vi "PLC ModbusTest.vi"() -> ()   [LabVIEW 2019]
uses:
  <vilib>/Plasmionique/MB Master/MB_Master_TCP/MB_Master_TCP.lvclass
  <vilib>/NI/Modbus Library/API/Wrapper/API Main.lvlib
  <vilib>/NI/Modbus Library/API/Master/Modbus Master.lvclass
  <vilib>/NI/Modbus Library/API/Wrapper/Create TCP Master.vi
panel:
  out "register values 3":u16[](array[numeric])
  out "remote port 2":u16
  out "remote address 2":string
  out "listener ID out":refnum<k5>
  out "remote port":u16
  out "remote address":string
  out "Words":i16[](array[numeric])
  out "Information out":T1 {"Unit identifier" max=247; "exceptionCode" max=247}
  out "error out 5":errorcluster
  out "register values 2":u16[](array[numeric])
  out "register values":u16[](array[numeric])
  out "error out 4":errorcluster
  out "Registers":u16[](array[numeric])
  out "concatenated string":string
  in  "Input ASCII":string="A"
  out "hex integer string":string
  in  "string":string="WR ZF0.H 41\r"
  out "value":i32
  out "ASCII Output":string
  out "error out 2":errorcluster
  out "data out 4":string
  out "data out 3":string
  in  "timeout ms (60000) 2":i32=6000
  out "data out":string
  in  "String":string="RDS DM0 4\r"
  out "error out":errorcluster
  in  "timeout ms (60000)":i32=6000
  # "Input ASCII"
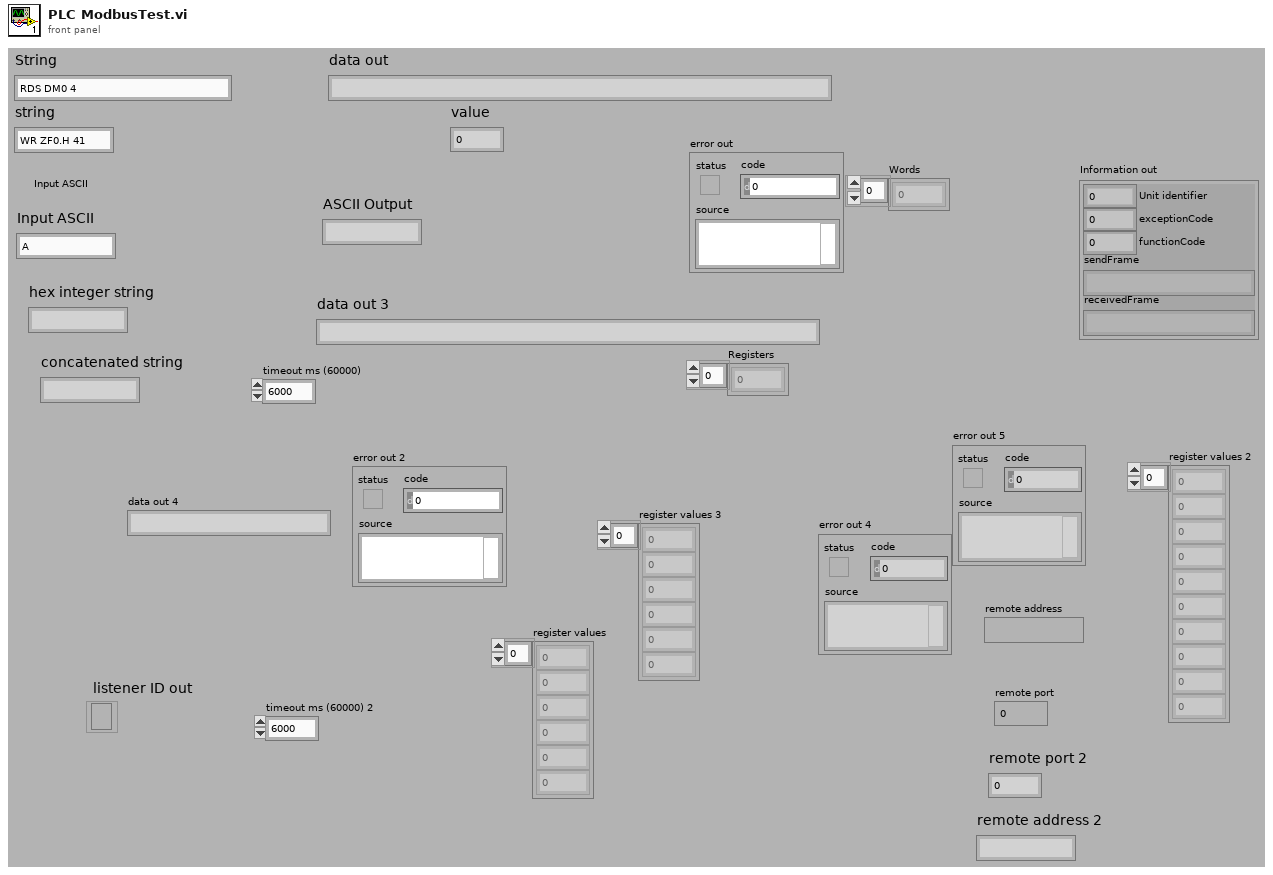
[diagram p1: front panel]
types:
  T1 = cluster{"Unit identifier":u8, "exceptionCode":u8, "functionCode":u8, "sendFrame":string, "receivedFrame":string}
  T2 = cluster{"server address":string, "remote port (502)":u16}
  T3 = enum16{"Standard", "Buffered", "CRLF", "Immediate"}
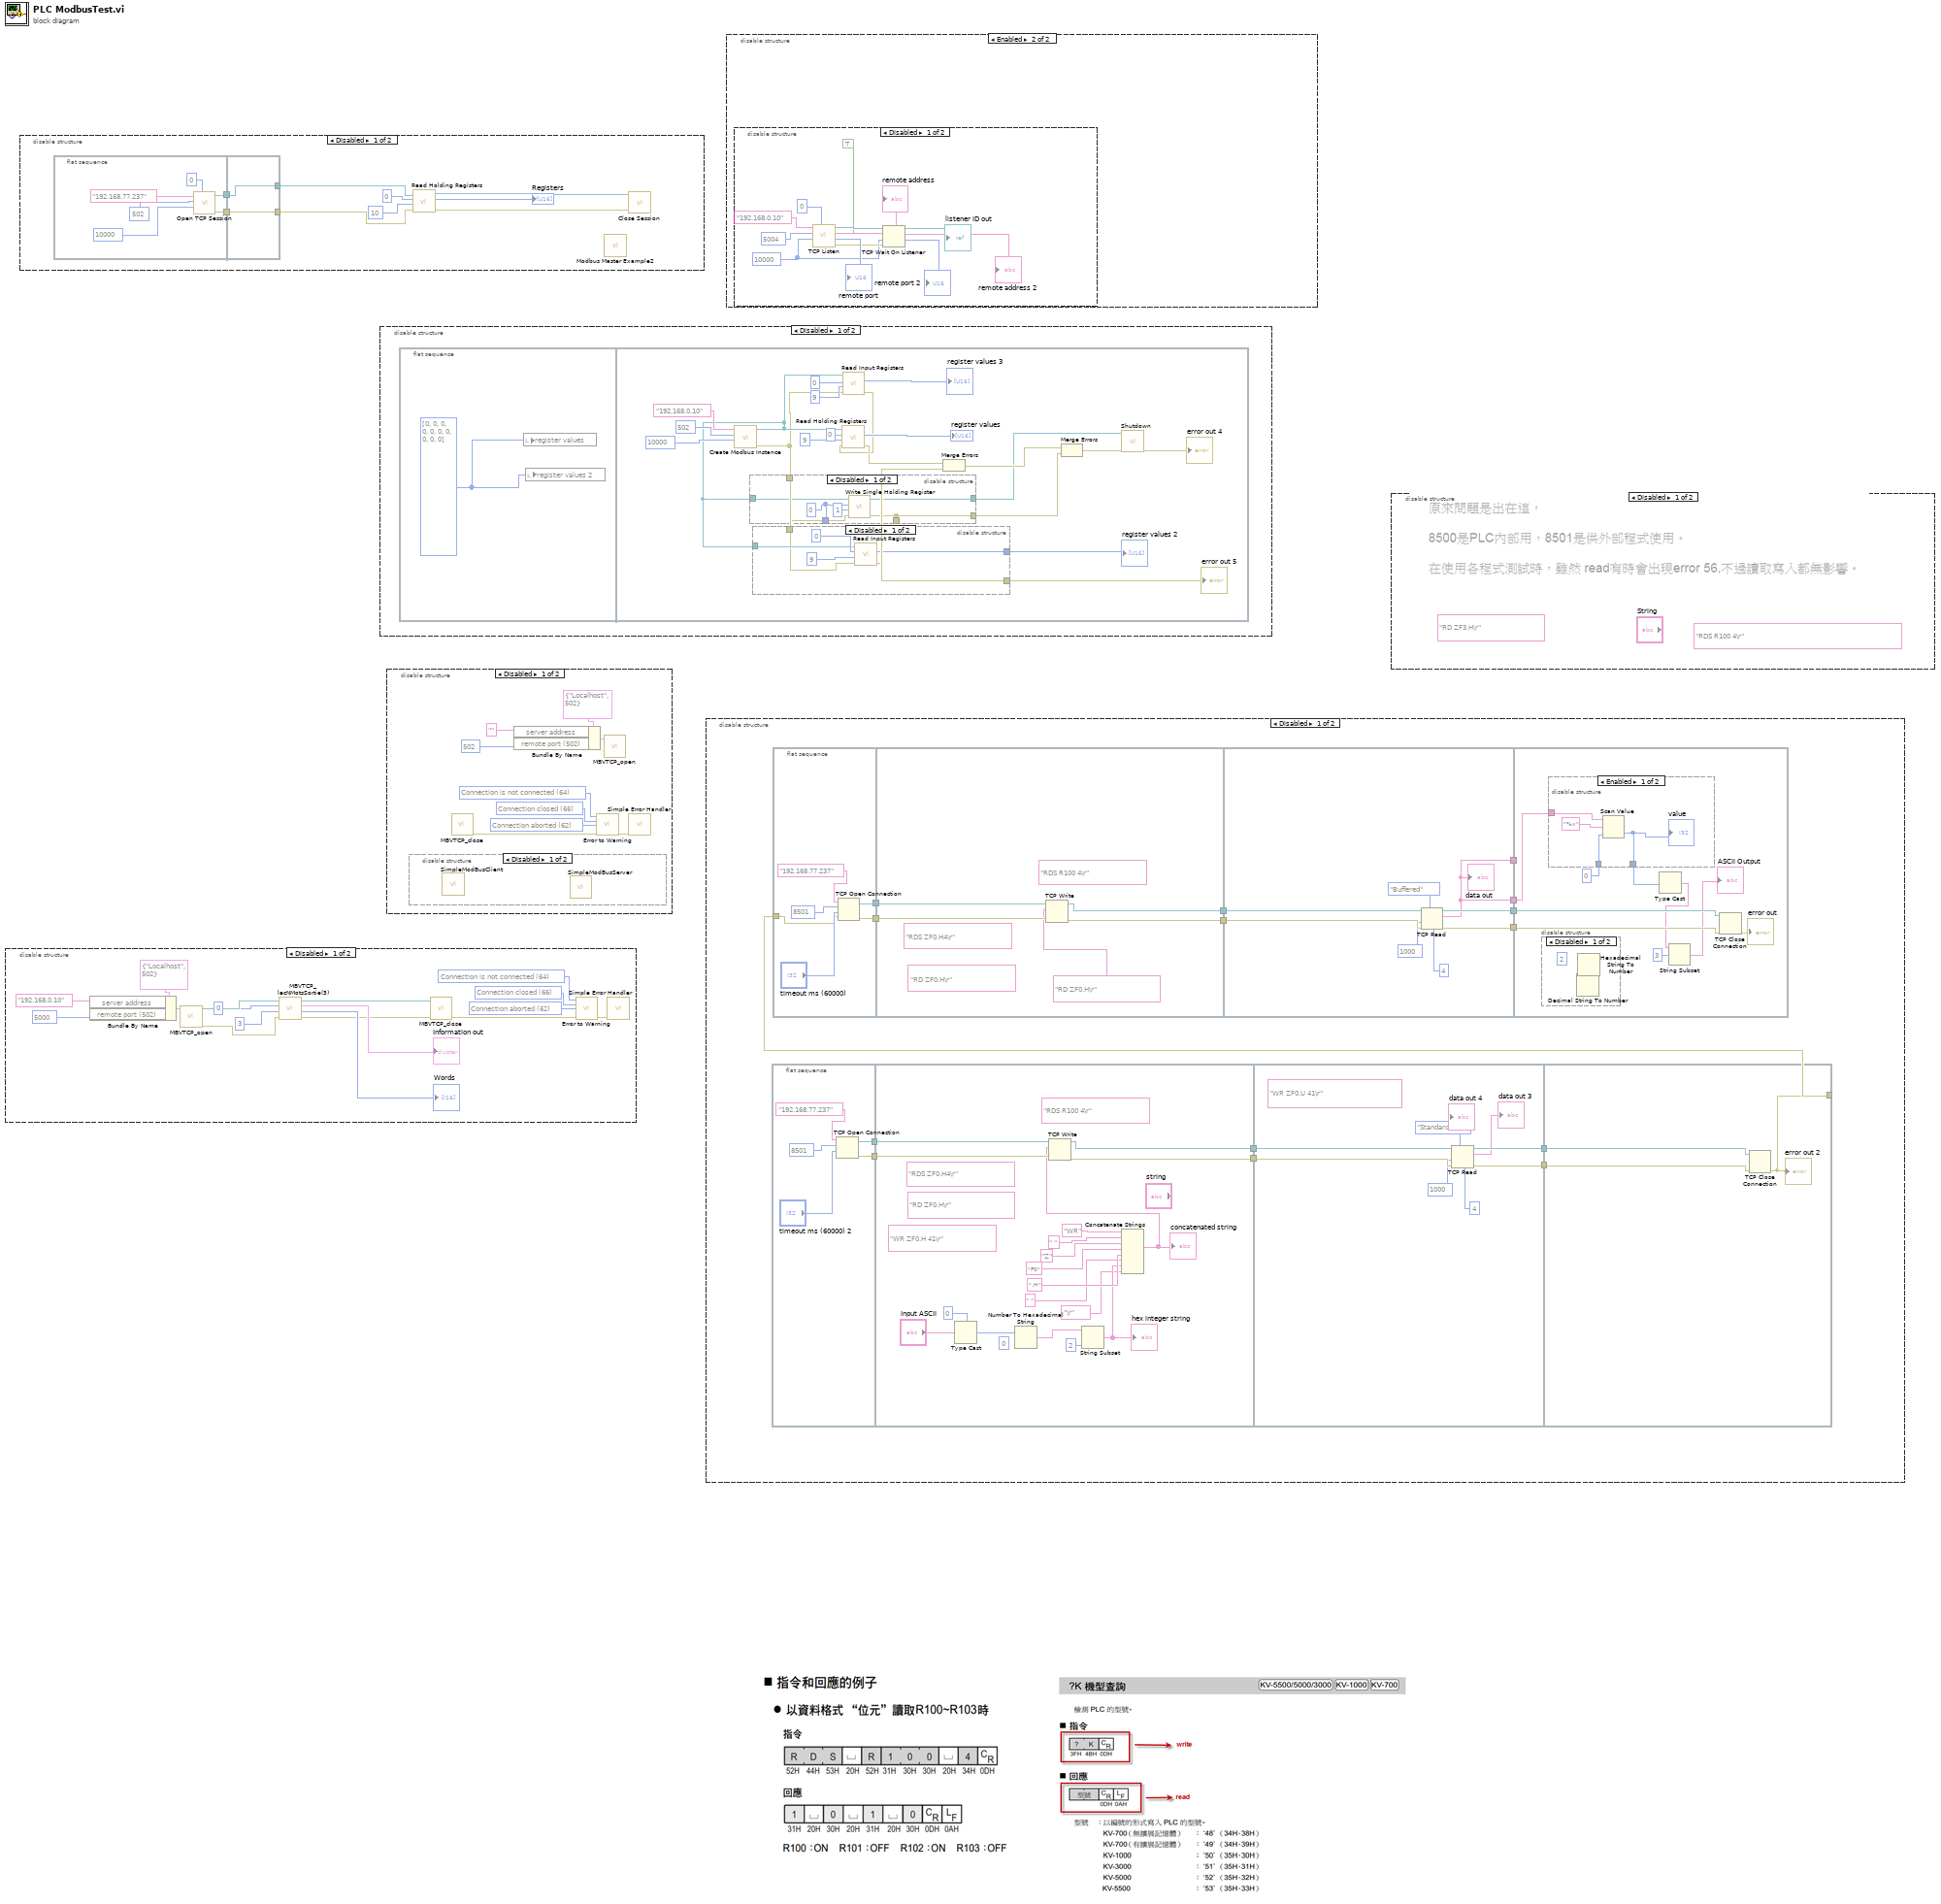
[diagram p0: block diagram]
diagram:
  n1 = disable-structure shown="Disabled" {
    frame Disabled {
      w10 = 62 items=["No Error", "Argument Error", "Memory Full", "Out of Zone", "End of File", "File Already Open", "Generic File IO Error", "File Not Found", "File Permission Error", "Disk Full", "Duplicate Path", "Too Many Files Open", "Not Enabled", "Resource File Not Found", "Cannot Add Resource", "Resource Not Found", "Image Not Found", "Image Memory Error", "Pen Does Not Exist", "Config Bad Type", "Config Token Not Found", "Config Parse Error", "Config Memory Error", "Bad External Code Format", "Bad External Code Offset", "External Code Not Present", "Null Window", "Destroy Window Mixup", "Null Menu", "Print Aborted", "Bad Print Record", "Print Driver Error", "Windows Error During Print", "Memory Error During Print", "Print Dialog Error", "Generic Print Error", "Invalid Device Refnum", "Device Not Found", "Device Parameter Error", "Device Unit Error", "Can't Open Device", "Device Call Aborted", "Generic Error", "Cancelled By User", "Object ID Too Low", "Object ID Too High", "Object Not In Heap", "Unknown Heap", "Bad DefProc ID", "DefProc Not In Table", "Message Out Of Range", "Null Method", "Unknown Message", "Manager Call Not Supported", "Bad address", "Connection In progress", "Connection timed out", "Connection is already in progress", "Network attribute not supported", "Network error", "Address in use", "System out of memory", "Connection aborted", "Connection refused", "Connection is not connected", "Connection is already connected", "Connection closed", "Initialize error (interapplication manager)", "Bad occurrence", "Wait on unbound occurrence handler", "Occurrence queue overflow", "Bad path", "Semaphore not signaled", "Unrecognized type (interapplication manager)"] ("1st Error to Convert")
      w11 = 66 items=["No Error", "Argument Error", "Memory Full", "Out of Zone", "End of File", "File Already Open", "Generic File IO Error", "File Not Found", "File Permission Error", "Disk Full", "Duplicate Path", "Too Many Files Open", "Not Enabled", "Resource File Not Found", "Cannot Add Resource", "Resource Not Found", "Image Not Found", "Image Memory Error", "Pen Does Not Exist", "Config Bad Type", "Config Token Not Found", "Config Parse Error", "Config Memory Error", "Bad External Code Format", "Bad External Code Offset", "External Code Not Present", "Null Window", "Destroy Window Mixup", "Null Menu", "Print Aborted", "Bad Print Record", "Print Driver Error", "Windows Error During Print", "Memory Error During Print", "Print Dialog Error", "Generic Print Error", "Invalid Device Refnum", "Device Not Found", "Device Parameter Error", "Device Unit Error", "Can't Open Device", "Device Call Aborted", "Generic Error", "Cancelled By User", "Object ID Too Low", "Object ID Too High", "Object Not In Heap", "Unknown Heap", "Bad DefProc ID", "DefProc Not In Table", "Message Out Of Range", "Null Method", "Unknown Message", "Manager Call Not Supported", "Bad address", "Connection In progress", "Connection timed out", "Connection is already in progress", "Network attribute not supported", "Network error", "Address in use", "System out of memory", "Connection aborted", "Connection refused", "Connection is not connected", "Connection is already connected", "Connection closed", "Initialize error (interapplication manager)", "Bad occurrence", "Wait on unbound occurrence handler", "Occurrence queue overflow", "Bad path", "Semaphore not signaled", "Unrecognized type (interapplication manager)"] ("1st Error to Convert")
      w12 = 64 items=["No Error", "Argument Error", "Memory Full", "Out of Zone", "End of File", "File Already Open", "Generic File IO Error", "File Not Found", "File Permission Error", "Disk Full", "Duplicate Path", "Too Many Files Open", "Not Enabled", "Resource File Not Found", "Cannot Add Resource", "Resource Not Found", "Image Not Found", "Image Memory Error", "Pen Does Not Exist", "Config Bad Type", "Config Token Not Found", "Config Parse Error", "Config Memory Error", "Bad External Code Format", "Bad External Code Offset", "External Code Not Present", "Null Window", "Destroy Window Mixup", "Null Menu", "Print Aborted", "Bad Print Record", "Print Driver Error", "Windows Error During Print", "Memory Error During Print", "Print Dialog Error", "Generic Print Error", "Invalid Device Refnum", "Device Not Found", "Device Parameter Error", "Device Unit Error", "Can't Open Device", "Device Call Aborted", "Generic Error", "Cancelled By User", "Object ID Too Low", "Object ID Too High", "Object Not In Heap", "Unknown Heap", "Bad DefProc ID", "DefProc Not In Table", "Message Out Of Range", "Null Method", "Unknown Message", "Manager Call Not Supported", "Bad address", "Connection In progress", "Connection timed out", "Connection is already in progress", "Network attribute not supported", "Network error", "Address in use", "System out of memory", "Connection aborted", "Connection refused", "Connection is not connected", "Connection is already connected", "Connection closed", "Initialize error (interapplication manager)", "Bad occurrence", "Wait on unbound occurrence handler", "Occurrence queue overflow", "Bad path", "Semaphore not signaled", "Unrecognized type (interapplication manager)"] ("1st Error to Convert")
      n2 = Bundle By Name(cluster=T2 {"server address"="Localhost", "remote port (502)"=502} ("Network"), "server address"="192.168.0.10" ("address"), "remote port (502)"=u16 5000) -> (w14:T2)
      n3 = call <vilib>:"MBVTCP_open.vi"("Network"=w14) -> ("error out"=w4:errorcluster, "NetRefTCP out"=w8:refnum<k5>)  [unwired: 2 in, 7 out]
      n4 = call <vilib>:"MBVTCP_lecNMotsSortie(3).vi"("error in"=w4, "Quantity of words (1)"=u16 3, "Word address"=u16 0, "NetRefTCP in"=w8) -> ("error out"=w1:errorcluster, "Words"=→"Words":i16[], "Information out"=→"Information out":T1, "NetRefTCP out"=w7:refnum<k5>)  [unwired: 4 in]
      n5 = call <vilib>:"MBVTCP_close.vi"("error in"=w1, "NetRefTCP in"=w7) -> ("error out"=w9:errorcluster)  [unwired: 9 out]
      n6 = call <vilib>:"Error to Warning.vi"("1st Error to Convert"=w12, "2nd Error to Convert"=w11, "3rd Error to Convert"=w10, "error in"=w9) -> ("warning out"=w13:errorcluster)  [unwired: 2 in, 9 out]
      n7 = call <vilib>:"Simple Error Handler.vi"("error in (no error)"=w13) -> ()  [unwired: 1 in, 8 out]
    }
    frame Enabled {
    }
  }
  n8 = disable-structure shown="Disabled" {
    frame Disabled {
      n9 = flat-sequence {
        tunnel: [w32] -> w26
        tunnel: [w27] -> w25
        tunnel: [w34] -> w22
        tunnel: w26 -> [w34]
        tunnel: w25 -> [w33]
        tunnel: [w33] -> w18
        frame #0 {
          n10 = call <vilib>:"Open TCP Session.vi"("Slave ID (255)"=0, "Timeout (10000)"=10000, "Port (502)"=u16 502 ("remote port (502)"), "IP Address"="192.168.77.237" ("address")) -> ("error out"=w32:errorcluster, "MB_TCP session"=w27:refnum<class "MB_Master_TCP.lvclass">)  [unwired: 6 in]
        }
        frame #1 {
        }
      }
      n11 = call <vilib>:"Read Holding Registers.vi"("error in (no error)"=w22, "quantity"=u16 10, "starting address"=u16 0, "MB session in"=w18) -> ("error out"=w19:errorcluster, "Registers"=→"Registers":u16[], "MB session out"=w20:refnum<class "MB_Master_TCP.lvclass">)  [unwired: 5 in]
      n12 = call <vilib>:"Modbus Master Example2.vi"() -> ()  [unwired: 8 in, 4 out]
      n13 = call-dynamic "Close Session.vi"("error in (no error)"=w19, "MB TCP session"=w20) -> ()  [unwired: 9 in, 1 out]
    }
    frame Enabled {
    }
  }
  n14 = disable-structure shown="Disabled" {
    frame Disabled {
      n15 = flat-sequence {
        frame #0 {
          w35 = u16[] [0, 0, 0, 0, 0, 0, 0, 0, 0, 0] ("register values 3")
          n16 = local write "register values"(w35) -> ()
          n17 = local write "register values 2"(w35) -> ()
        }
        frame #1 {
          n18 = call-poly <vilib>:"Create Modbus Instance.vi"("connect timeout ms"=10000, "port (502)"=u16 502 ("remote port (502)"), "address"="192.168.0.10") -> ("error out"=w37:errorcluster, "TCP master instance"=w40:refnum<class "Modbus Master.lvclass">)  [unwired: 7 in]
          n19 = disable-structure shown="Disabled" {
            disable-tunnel: w40 -> [w66 _]
            disable-tunnel: [w65 _] -> _
            disable-tunnel: w37 -> [w64 _]
            disable-tunnel: [w63 _] -> _
            disable-tunnel: [w63 _] -> w47
            disable-tunnel: [w62 _] -> w46
            frame Disabled {
              w65 = u16 0 ("starting address")
              n20 = call-dynamic "Write Single Holding Register.vi"("error in"=w64, "register to write"=u16 1, "address"=w65, "Modbus master in"=w66) -> ("error out"=w63:errorcluster, "Modbus master out"=w62:refnum<class "Modbus Master.lvclass">)  [unwired: 6 in]
            }
            frame Enabled {
            }
          }
          n21 = disable-structure shown="Disabled" {
            disable-tunnel: [w60 _] -> w51
            disable-tunnel: [w59 _] -> w50
            disable-tunnel: w40 -> [w57 _]
            disable-tunnel: w37 -> [w56 _]
            frame Disabled {
              n22 = call-dynamic "Read Input Registers.vi"("error in"=w56, "number of inputs"=u16 9, "starting address"=u16 0 ("number of inputs"), "Modbus master in"=w57) -> ("error out"=w60:errorcluster, "register values"=w59:u16[])  [unwired: 5 in, 1 out]
            }
            frame Enabled {
            }
          }
          "register values 2" <- w50
          "error out 5" <- w51
          n23 = call-dynamic "Read Input Registers.vi"("error in"=w37, "number of inputs"=u16 9 ("starting address"), "starting address"=u16 0, "Modbus master in"=w40) -> ("error out"=w36:errorcluster, "register values"=→"register values 3":u16[])  [unwired: 5 in, 1 out]
          n24 = call-dynamic <vilib>:"Read Holding Registers.vi"("error in"=w36, "number of inputs"=u16 9 ("starting address"), "starting address"=u16 0, "Modbus master in"=w40) -> ("error out"=w42:errorcluster, "register values"=→"register values":u16[])  [unwired: 5 in, 1 out]
          n25 = Merge Errors(w42, w51) -> (w49:errorcluster)
          n26 = Merge Errors(w49, w47) -> (w48:errorcluster)
          n27 = call-dynamic "Shutdown.vi"("error in"=w48, "Modbus master in"=w46) -> ("error out"=→"error out 4":errorcluster)  [unwired: 9 in]
        }
      }
    }
    frame Enabled {
    }
  }
  n28 = disable-structure shown="Disabled" {
    frame Disabled {
      w73 = 62 items=["No Error", "Argument Error", "Memory Full", "Out of Zone", "End of File", "File Already Open", "Generic File IO Error", "File Not Found", "File Permission Error", "Disk Full", "Duplicate Path", "Too Many Files Open", "Not Enabled", "Resource File Not Found", "Cannot Add Resource", "Resource Not Found", "Image Not Found", "Image Memory Error", "Pen Does Not Exist", "Config Bad Type", "Config Token Not Found", "Config Parse Error", "Config Memory Error", "Bad External Code Format", "Bad External Code Offset", "External Code Not Present", "Null Window", "Destroy Window Mixup", "Null Menu", "Print Aborted", "Bad Print Record", "Print Driver Error", "Windows Error During Print", "Memory Error During Print", "Print Dialog Error", "Generic Print Error", "Invalid Device Refnum", "Device Not Found", "Device Parameter Error", "Device Unit Error", "Can't Open Device", "Device Call Aborted", "Generic Error", "Cancelled By User", "Object ID Too Low", "Object ID Too High", "Object Not In Heap", "Unknown Heap", "Bad DefProc ID", "DefProc Not In Table", "Message Out Of Range", "Null Method", "Unknown Message", "Manager Call Not Supported", "Bad address", "Connection In progress", "Connection timed out", "Connection is already in progress", "Network attribute not supported", "Network error", "Address in use", "System out of memory", "Connection aborted", "Connection refused", "Connection is not connected", "Connection is already connected", "Connection closed", "Initialize error (interapplication manager)", "Bad occurrence", "Wait on unbound occurrence handler", "Occurrence queue overflow", "Bad path", "Semaphore not signaled", "Unrecognized type (interapplication manager)"] ("1st Error to Convert")
      w72 = 66 items=["No Error", "Argument Error", "Memory Full", "Out of Zone", "End of File", "File Already Open", "Generic File IO Error", "File Not Found", "File Permission Error", "Disk Full", "Duplicate Path", "Too Many Files Open", "Not Enabled", "Resource File Not Found", "Cannot Add Resource", "Resource Not Found", "Image Not Found", "Image Memory Error", "Pen Does Not Exist", "Config Bad Type", "Config Token Not Found", "Config Parse Error", "Config Memory Error", "Bad External Code Format", "Bad External Code Offset", "External Code Not Present", "Null Window", "Destroy Window Mixup", "Null Menu", "Print Aborted", "Bad Print Record", "Print Driver Error", "Windows Error During Print", "Memory Error During Print", "Print Dialog Error", "Generic Print Error", "Invalid Device Refnum", "Device Not Found", "Device Parameter Error", "Device Unit Error", "Can't Open Device", "Device Call Aborted", "Generic Error", "Cancelled By User", "Object ID Too Low", "Object ID Too High", "Object Not In Heap", "Unknown Heap", "Bad DefProc ID", "DefProc Not In Table", "Message Out Of Range", "Null Method", "Unknown Message", "Manager Call Not Supported", "Bad address", "Connection In progress", "Connection timed out", "Connection is already in progress", "Network attribute not supported", "Network error", "Address in use", "System out of memory", "Connection aborted", "Connection refused", "Connection is not connected", "Connection is already connected", "Connection closed", "Initialize error (interapplication manager)", "Bad occurrence", "Wait on unbound occurrence handler", "Occurrence queue overflow", "Bad path", "Semaphore not signaled", "Unrecognized type (interapplication manager)"] ("1st Error to Convert")
      w71 = 64 items=["No Error", "Argument Error", "Memory Full", "Out of Zone", "End of File", "File Already Open", "Generic File IO Error", "File Not Found", "File Permission Error", "Disk Full", "Duplicate Path", "Too Many Files Open", "Not Enabled", "Resource File Not Found", "Cannot Add Resource", "Resource Not Found", "Image Not Found", "Image Memory Error", "Pen Does Not Exist", "Config Bad Type", "Config Token Not Found", "Config Parse Error", "Config Memory Error", "Bad External Code Format", "Bad External Code Offset", "External Code Not Present", "Null Window", "Destroy Window Mixup", "Null Menu", "Print Aborted", "Bad Print Record", "Print Driver Error", "Windows Error During Print", "Memory Error During Print", "Print Dialog Error", "Generic Print Error", "Invalid Device Refnum", "Device Not Found", "Device Parameter Error", "Device Unit Error", "Can't Open Device", "Device Call Aborted", "Generic Error", "Cancelled By User", "Object ID Too Low", "Object ID Too High", "Object Not In Heap", "Unknown Heap", "Bad DefProc ID", "DefProc Not In Table", "Message Out Of Range", "Null Method", "Unknown Message", "Manager Call Not Supported", "Bad address", "Connection In progress", "Connection timed out", "Connection is already in progress", "Network attribute not supported", "Network error", "Address in use", "System out of memory", "Connection aborted", "Connection refused", "Connection is not connected", "Connection is already connected", "Connection closed", "Initialize error (interapplication manager)", "Bad occurrence", "Wait on unbound occurrence handler", "Occurrence queue overflow", "Bad path", "Semaphore not signaled", "Unrecognized type (interapplication manager)"] ("1st Error to Convert")
      n29 = disable-structure shown="Disabled" {
        frame Disabled {
          n30 = call "SimpleModBusClient.vi"() -> ()  [unwired: 1 in]
          n31 = call "SimpleModBusServer.vi"() -> ()  [unwired: 12 in]
        }
        frame Enabled {
        }
      }
      n32 = call <vilib>:"MBVTCP_close.vi"() -> ("error out"=w74:errorcluster)  [unwired: 2 in, 9 out]
      n33 = Bundle By Name(cluster=T2 {"server address"="Localhost", "remote port (502)"=502} ("Network"), "server address"="" ("address"), "remote port (502)"=u16 502) -> (w76:T2)
      n34 = call <vilib>:"Error to Warning.vi"("1st Error to Convert"=w71, "2nd Error to Convert"=w72, "3rd Error to Convert"=w73, "error in"=w74) -> ("warning out"=w70:errorcluster)  [unwired: 2 in, 9 out]
      n35 = call <vilib>:"MBVTCP_open.vi"("Network"=w76) -> ()  [unwired: 2 in, 9 out]
      n36 = call <vilib>:"Simple Error Handler.vi"("error in (no error)"=w70) -> ()  [unwired: 1 in, 8 out]
    }
    frame Enabled {
    }
  }
  n37 = disable-structure shown="Disabled" {
    frame Disabled {
      n38 = flat-sequence {
        tunnel: [w95] -> w83
        tunnel: [w94] -> w82
        tunnel: w83 -> [w114]
        tunnel: [w113] -> w81
        tunnel: w82 -> [w112]
        tunnel: [w111] -> w80
        tunnel: w81 -> [w122]
        tunnel: w80 -> [w121]
        tunnel: [w119] -> w79
        tunnel: [w118] -> w78
        tunnel: w79 -> [w125]
        tunnel: w78 -> [w124]
        tunnel: [w123] -> w77
        frame #0 {
          n39 = TCP Open Connection(address="192.168.77.237", remote port or service name=u32 8501 ("remote port"), timeout ms (60000)="timeout ms (60000) 2") -> (connection ID=w95:refnum<k5>, error out=w94:errorcluster)  [unwired: 2 in]
        }
        frame #1 {
          (unwired) i16 0 ("width (-)")
          (unwired) "WR ZF0.H 41\r" ("string")
          (unwired) "RDS ZF0.H4\r" ("string")
          (unwired) "RD ZF0.H\r" ("string")
          (unwired) "RDS R100 4\r" ("string")
          n40 = Type Cast(type=0, x="Input ASCII") -> (*(type *) &x=w107:i32)
          n41 = Number To Hexadecimal String(2:w107) -> (0:w102:string)  [unwired: 1 in]
          n42 = String Subset(string=w102, length (rest)=2) -> (substring=w99:string)  [unwired: 1 in]
          "hex integer string" <- w99
          n43 = Concatenate Strings("WR", " ", "Z", "F0", ".H", " ", w99, "\r") -> (w103:string)
          "concatenated string" <- w103
          n44 = TCP Write(connection ID=w114, data in=w103, error in (no error)=w112) -> (connection ID out=w113:refnum<k5>, error out=w111:errorcluster)  [unwired: 1 in, 1 out]
        }
        frame #2 {
          (unwired) "WR ZF0.U 41\r"
          n45 = TCP Read(connection ID=w122, bytes to read=4, error in (no error)=w121, 7:T3."Standard" ("mode (standard)"), 9:1000 ("timeout ms (25000)")) -> (connection ID out=w119:refnum<k5>, data out=→"data out 3":string, error out=w118:errorcluster)
        }
        frame #3 {
          n46 = TCP Close Connection(connection ID=w125, error in (no error)=w124) -> (error out=w123:errorcluster)  [unwired: 1 in, 1 out]
          "error out 2" <- w123
        }
      }
      n47 = flat-sequence {
        tunnel: [w130] -> w91
        tunnel: [w129] -> w90
        tunnel: w77 -> [w126]
        tunnel: w91 -> [w136]
        tunnel: [w135] -> w89
        tunnel: w90 -> [w134]
        tunnel: [w133] -> w88
        tunnel: w89 -> [w144]
        tunnel: w88 -> [w143]
        tunnel: [w141] -> w87
        tunnel: [w140] -> w86
        tunnel: [w137] -> w85
        tunnel: [w137] -> w84
        tunnel: w87 -> [w153]
        tunnel: w86 -> [w152]
        tunnel: w85 -> [_]
        tunnel: w84 -> [w150]
        frame #0 {
          n48 = TCP Open Connection(address="192.168.77.237", remote port or service name=u32 8501 ("remote port"), timeout ms (60000)="timeout ms (60000)", error in (no error)=w126) -> (connection ID=w130:refnum<k5>, error out=w129:errorcluster)  [unwired: 1 in]
        }
        frame #1 {
          (unwired) "RDS ZF0.H4\r" ("string")
          (unwired) "RD ZF0.H\r" ("string")
          (unwired) "RDS R100 4\r" ("string")
          n49 = TCP Write(connection ID=w136, data in="RD ZF0.H\r" ("string"), error in (no error)=w134) -> (connection ID out=w135:refnum<k5>, error out=w133:errorcluster)  [unwired: 1 in, 1 out]
        }
        frame #2 {
          n50 = TCP Read(connection ID=w144, bytes to read=4, error in (no error)=w143, 7:T3."Buffered" ("mode (standard)"), 9:1000 ("timeout ms (25000)")) -> (connection ID out=w141:refnum<k5>, data out=w137:string, error out=w140:errorcluster)
          "data out" <- w137
        }
        frame #3 {
          n51 = disable-structure shown="Disabled" {
            frame Disabled {
              (unwired) 2 ("offset")
              n52 = Decimal String To Number() -> ()  [unwired: 3 in, 2 out]
              n53 = Hexadecimal String To Number() -> ()  [unwired: 3 in, 2 out]
            }
            frame Enabled {
            }
          }
          n54 = disable-structure shown="Enabled" {
            disable-tunnel: w150 -> [w156 _]
            disable-tunnel: [w155 _] -> w145
            disable-tunnel: 0 -> [w154 _]
            frame Enabled {
              n55 = Scan Value(string=w156, format string="%x", default (0 dbl)=w154) -> (value=w155:i32)  [unwired: 1 out]
              "value" <- w155
            }
            frame Disabled {
            }
          }
          n56 = Type Cast(x=w145) -> (*(type *) &x=w147:string)  [unwired: 1 in]
          n57 = String Subset(string=w147, offset (0)=3) -> (substring=→"ASCII Output":string)  [unwired: 1 in]
          n58 = TCP Close Connection(connection ID=w153, error in (no error)=w152) -> (error out=→"error out":errorcluster)  [unwired: 1 in, 1 out]
        }
      }
    }
    frame Enabled {
    }
  }
  n59 = disable-structure shown="Enabled" {
    frame Disabled {
    }
    frame Enabled {
      n60 = disable-structure shown="Disabled" {
        frame Disabled {
          w163 = 10000 ("connect timeout ms")
          n61 = call <vilib>:"TCP Listen.vi"("net address"=u32 0, "timeout ms (wait forever: -1)"=w163, "port"=u16 5004 ("remote port (502)"), "service name"="192.168.0.10" ("address")) -> ("error out"=w164:errorcluster, "remote port"=→"remote port":u16, "remote address"=→"remote address":string, "connection ID"=w167:refnum<k5>)  [unwired: 3 in, 1 out]
          n62 = TCP Wait On Listener(8:w164, 9:w163, 10:TRUE ("resolve remote address (T)"), 11:w167) -> (1:→"remote port 2":u16, 2:→"remote address 2":string, 3:→"listener ID out":refnum<k5>)  [unwired: 2 out]
        }
        frame Enabled {
        }
      }
    }
  }
  n63 = disable-structure shown="Disabled" {
    frame Disabled {
      (unwired) "RD ZF3.H\r" ("string")
      (unwired) "RDS R100 4\r" ("string")
    }
    frame Enabled {
    }
  }
